vi "Write userEventPeriod.vi"(8 "error in (no error)":errorcluster, 10 "userEventPeriod":refnum<user-event>, 11 "WindowsTarget in":refnum<class "cRIOScanModeTarget.lvclass">) -> (0 "error out":errorcluster, 3 "WindowsTarget out":refnum<class "cRIOScanModeTarget.lvclass">)   [LabVIEW 2012, in "cRIOScanModeTarget.lvclass"]
uses:
  cRIOScanModeTarget.lvclass
  cRIOScanModeTarget.lvclass/cRIOScanModeTarget.ctl
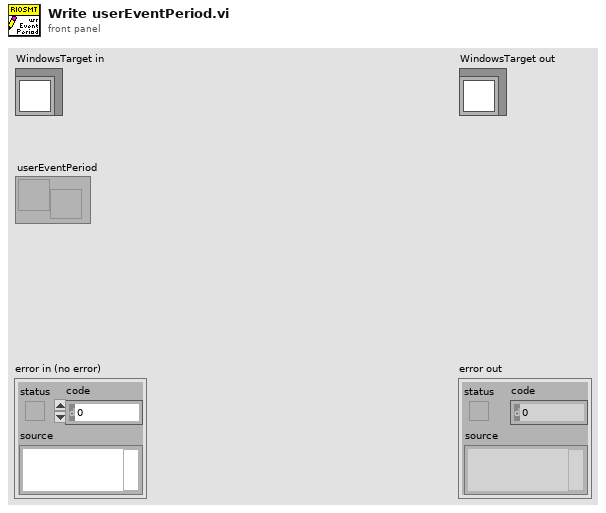
[diagram p1: front panel]
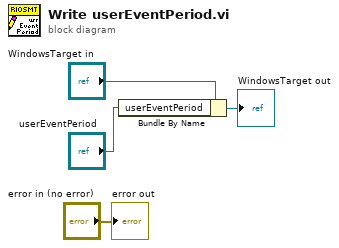
[diagram p0: block diagram]
diagram:
  n1 = Bundle By Name(cluster="WindowsTarget in", "userEventPeriod"="userEventPeriod") -> (→"WindowsTarget out":refnum<class "cRIOScanModeTarget.lvclass">)
  "error out" <- "error in (no error)"
